vi "בדיקת מתח תפיסה של סליל פיקוד ללא עומס 4.vi"(8 "error":errorcluster, 11 "Path for Log":path) -> (0 "error out":errorcluster, 1 "מצב ממסר פתוח/סגור":bool, 2 "מתח סגירת הממסר":dbl format="%.4f", 3 "מתח מוצא מהספק":dbl format="%.4f", 5 "resultUserPrompt":bool)   [LabVIEW 2015]
uses:
  <vilib>/DAQmx/write.llb/DAQmx Write (Digital Bool 1Line 1Point).vi
  <vilib>/DAQmx/create/channels.llb/DAQmx Create Channel (DO-Digital Output).vi
  <vilib>/DAQmx/miscellaneous.llb/DAQmx Fill In Error Info.vi
panel:
  out "progress":dbl(slide) scale=0.0..36.0
  out "error IO DMM":errorcluster
  in  "Stop Button":bool
  # "Right-Click to\nexplain error"
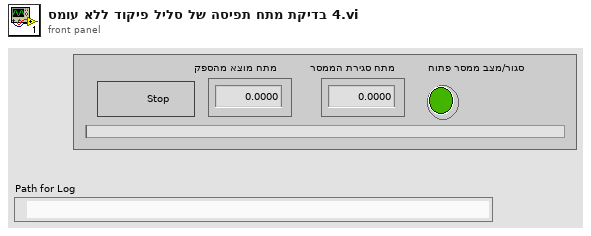
[diagram p1: front panel]
types:
  T1 = enum32{"Invalid", "Standard", "Closed", "Hidden", "Minimized", "Maximized"}
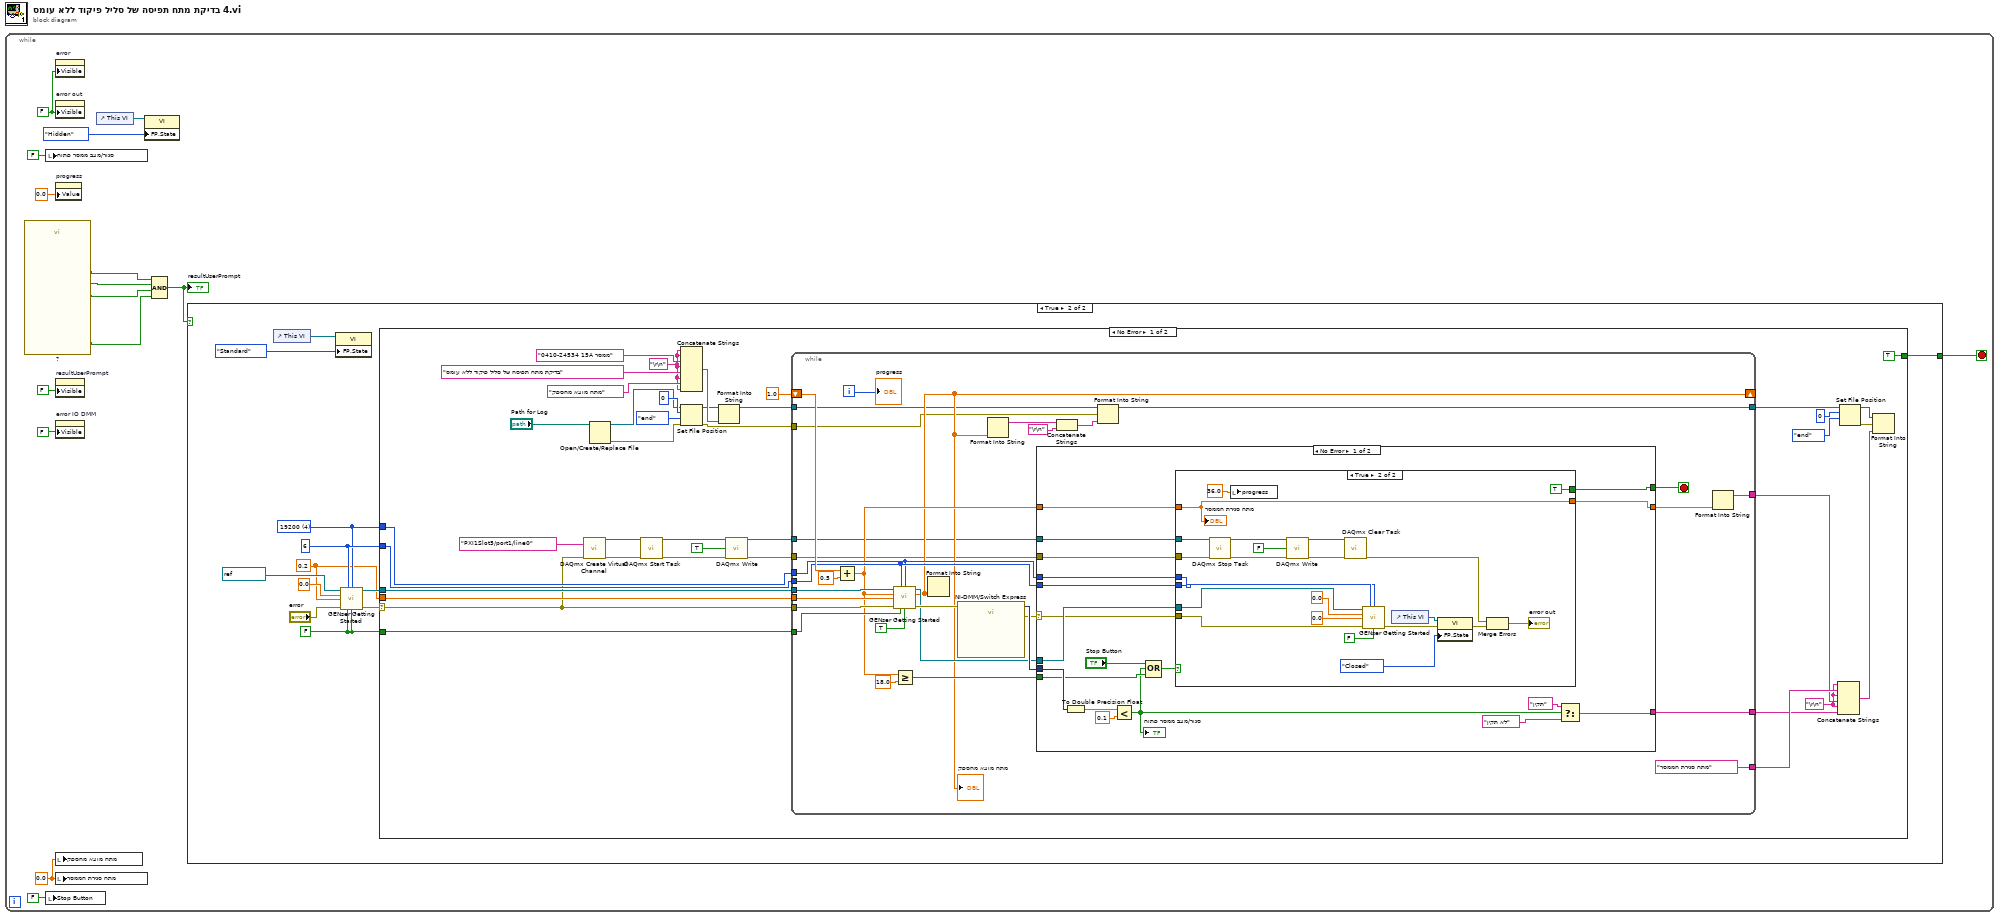
[diagram p0: block diagram]
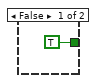
[diagram p2: hidden frame]
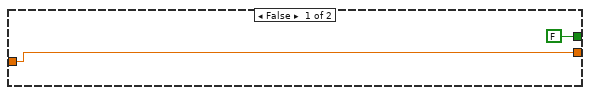
[diagram p3: hidden frame]
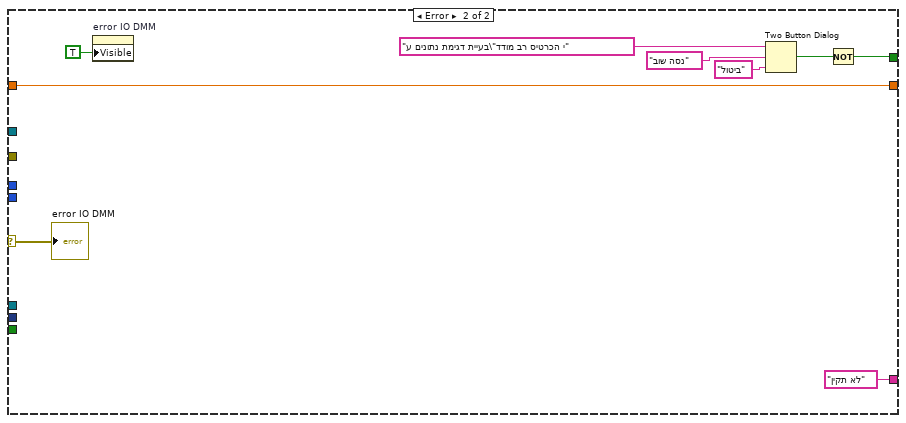
[diagram p4: hidden frame]
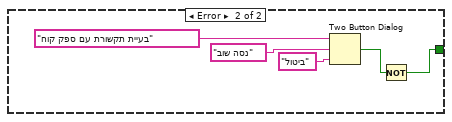
[diagram p5: hidden frame]
diagram:
  n1 = while {
    stop <- w1 stop-if-true
    w7 = FALSE ("Visible")
    w10 = 0.0 ("signals out")
    n2 = call "?"() -> ("הדקי הרב מודד"=w2:bool, "(מגע שלילי (מעטפת"=w3:bool, "A מגע חיובי"=w4:bool, "OK"=w5:bool)  [unwired: 15 in, 1 out]
    n3 = local write "מצב ממסר פתוח/סגור"(FALSE ("מגע סגור")) -> ()
    n4 = local write "Stop Button"(FALSE ("Reset (T)")) -> ()
    n5 = property on="error" class="Clust (strict)"("Visible"=w7) -> ()  [unwired: 2 in, 2 out]
    n6 = property on="error out" class="Clust (strict)"("Visible"=w7) -> ()  [unwired: 2 in, 2 out]
    n7 = property on="progress" class="Slide (strict)"("Value"=0.0 ("progress")) -> ()  [unwired: 2 in, 2 out]
    n8 = property on="resultUserPrompt" class="Bool (strict)"("Visible"=FALSE) -> ()  [unwired: 2 in, 2 out]
    n9 = property on="error IO DMM" class="Clust (strict)"("Visible"=FALSE) -> ()  [unwired: 2 in, 2 out]
    n10 = local write "מתח מוצא מהספק"(w10) -> ()
    n11 = local write "מתח סגירת הממסר"(w10) -> ()
    n12 = control-ref of="This VI"() -> (w9:refnum<vi>)
    n13 = property class="VI"(reference=w9, "FP.State"=T1."Hidden" ("Front Panel Window:State")) -> ()  [unwired: 1 in, 2 out]
    n14 = Compound Arithmetic op=AND(w5, w4, w3, w2) -> (w15:bool)
    "resultUserPrompt" <- w15
    n15 = case shown="True" w15 {
      tunnel: [TRUE ("T button?") w22] -> w1
      frame False {
      }
      frame True {
        w21 = FALSE ("Output On (T)")
        w26 = u16 4 items=["1200", "2400", "4800", "9600", "19200"] ("BAUD")
        w27 = i16 6 ("GEN Addr")
        w23 = 0.2 ("Current Limit")
        n16 = control-ref of="This VI"() -> (w19:refnum<vi>)
        n17 = property class="VI"(reference=w19, "FP.State"=T1."Standard" ("Front Panel Window:State")) -> ()  [unwired: 1 in, 2 out]
        n18 = call "GENser Getting Started.vi"("VISA"=refnum<visa-resource-name> "COM6", "GEN Addr"=w27, "BAUD"=w26, "Voltage Limit"=0.0, "Current Limit"=w23, "error"="error", "Reset (T)"=w21, "Output On (T)"=w21) -> ("VISA out"=w28:refnum<visa-resource-name>, "error out"=w18:errorcluster)  [unwired: 4 in, 2 out]
        n19 = case shown="No Error" w18 {
          selector: w18 -> [w29 _]
          tunnel: w28 -> [w67 _]
          tunnel: w27 -> [w66 _]
          tunnel: w26 -> [w65 _]
          tunnel: w21 -> [w64 _]
          tunnel: w23 -> [w63 _]
          tunnel: [TRUE w152] -> w22
          frame No Error {
            w38 = "\r\n"
            w57 = "\r\n"
            n20 = call-poly <vilib>:"DAQmx Create Virtual Channel.vi"("lines"=tag "PXI1Slot5/port1/line0", "error in"=w29) -> ("task out"=w36:refnum<k21>, "error out"=w37:errorcluster)  [unwired: 12 in]
            n21 = Open/Create/Replace File(file path (use dialog)="Path for Log") -> (refnum out=w48:refnum<file>, error out=w47:errorcluster)  [unwired: 5 in, 1 out]
            n22 = call <vilib>:"DAQmx Start Task.vi"("task/channels in"=w36, "error in"=w37) -> ("task out"=w33:refnum<k21>, "error out"=w32:errorcluster)  [unwired: 12 in]
            n23 = Concatenate Strings(w38, w38, "0410-24534 15A ממסר", w38, "בדיקת מתח תפיסה של סליל פיקוד ללא עומס", w38, "מתח מוצא מהספק", w38) -> (w44:string)
            n24 = Set File Position(offset (in bytes) (0)=i64 0, refnum=w48, from (0:start)=enum16{"start", "end", "current"}."end", error in=w47) -> (refnum out=w40:refnum<file>, error out=w45:errorcluster)
            n25 = Format Into String(initial string=w40, w44) -> (resulting string=w39:refnum<file>)  [unwired: 2 in, 1 out]
            n26 = call-poly <vilib>:"DAQmx Write.vi"("task/channels in"=w33, "data"=TRUE, "error in"=w32) -> ("task out"=w31:refnum<k21>, "error out"=w30:errorcluster)  [unwired: 10 in, 1 out]
            n27 = while {
              tunnel: w67 -> [w87]
              tunnel: w29 -> [w98]
              tunnel: w66 -> [w89]
              tunnel: w65 -> [w88]
              tunnel: w64 -> [w97]
              tunnel: w63 -> [w95]
              shift-right: [w79] -> _
              shift-left: 1.0 ("y") -> [w93]
              tunnel: ["מתח סגירת הממסר"] -> w60
              tunnel: [w77] -> w59
              tunnel: [w76] -> w58
              tunnel: [w73] -> w56
              tunnel: w39 -> [w72]
              tunnel: w45 -> [w71]
              tunnel: w31 -> [w69]
              tunnel: w30 -> [w68]
              i -> [w80]
              stop <- w90 stop-if-true
              n28 = Add(x=w93, y=0.5) -> (x+y=w81:dbl)
              n29 = call "GENser Getting Started.vi"("VISA"=w87, "GEN Addr"=w89, "BAUD"=w88, "Voltage Limit"=w81, "Current Limit"=w95, "error"=w98, "Reset (T)"=w97, "Output On (T)"=TRUE) -> ("VISA out"=w86:refnum<visa-resource-name>, "Output Voltage"=w79:dbl, "error out"=w92:errorcluster)  [unwired: 4 in, 1 out]
              "מתח מוצא מהספק" <- w79
              n30 = Greater Or Equal?(x=w81, y=18.0) -> (x >= y?=w84:bool)
              n31 = Format Into String(w79) -> ()  [unwired: 3 in, 2 out]
              n32 = call "NI-DMM/Switch Express"("error in"=w92) -> ("signals out"=w91:dynamicdata, "error out"=w83:errorcluster)  [unwired: 16 in, 1 out]
              n33 = Format Into String(w79) -> (resulting string=w74:string)  [unwired: 3 in, 1 out]
              n34 = case shown="No Error" w83 {
                selector: w83 -> [w109 w151]
                tunnel: w91 -> [w117 _]
                tunnel: [w106 w143] -> w90
                tunnel: w89 -> [w114 _]
                tunnel: w88 -> [w113 _]
                tunnel: w86 -> [w112 _]
                tunnel: w84 -> [w111 _]
                tunnel: w81 -> [w110 w146]
                tunnel: [w105 w146] -> w82
                tunnel: [w102 "לא תקין"] -> w76
                tunnel: w69 -> [w100 _]
                tunnel: w68 -> [w99 _]
                frame No Error {
                  n35 = To Double Precision Float(number=w117) -> (double precision float=w108:dbl)
                  n36 = Less?(x=w108, y=0.1) -> (x < y?=w101:bool)
                  "מצב ממסר פתוח/סגור" <- w101
                  n37 = Compound Arithmetic op=OR("Stop Button", w101, w111) -> (w116:bool)
                  n38 = case shown="True" w116 {
                    tunnel: [FALSE TRUE] -> w106
                    tunnel: w114 -> [_ w142]
                    tunnel: w113 -> [_ w141]
                    tunnel: w112 -> [_ w140]
                    tunnel: w109 -> [_ w137]
                    tunnel: w110 -> [w118 w132]
                    tunnel: [w118 w132] -> w105
                    tunnel: w100 -> [_ w122]
                    tunnel: w99 -> [_ w121]
                    frame False {
                    }
                    frame True {
                      n39 = call <vilib>:"DAQmx Stop Task.vi"("task/channels in"=w122, "error in"=w121) -> ("task out"=w130:refnum<k21>, "error out"=w128:errorcluster)  [unwired: 12 in]
                      n40 = local write "progress"(36.0 ("progress")) -> ()
                      n41 = call-poly <vilib>:"DAQmx Write.vi"("task/channels in"=w130, "data"=FALSE, "error in"=w128) -> ("task out"=w127:refnum<k21>, "error out"=w126:errorcluster)  [unwired: 10 in, 1 out]
                      n42 = call <vilib>:"DAQmx Clear Task.vi"("task in"=w127, "error in"=w126) -> ("error out"=w123:errorcluster)  [unwired: 13 in]
                      n43 = call "GENser Getting Started.vi"("VISA"=w140, "GEN Addr"=w142, "BAUD"=w141, "Voltage Limit"=0.0, "Current Limit"=0.0, "error"=w137, "Output On (T)"=FALSE) -> ("error out"=w120:errorcluster)  [unwired: 5 in, 3 out]
                      n44 = control-ref of="This VI"() -> (w134:refnum<vi>)
                      n45 = property class="VI"(reference=w134, error in=w120, "FP.State"=T1."Closed" ("Front Panel Window:State")) -> (error out=w124:errorcluster)  [unwired: 1 out]
                      n46 = Merge Errors(w123, w124) -> (→"error out":errorcluster)
                      "מתח סגירת הממסר" <- w132
                    }
                  }
                  n47 = Select(t="תקין", s=w101, f="לא תקין") -> (s? t:f=w102:string)
                }
                frame Error {
                  n48 = property on="error IO DMM" class="Clust (strict)"("Visible"=TRUE) -> ()  [unwired: 2 in, 2 out]
                  n49 = Two Button Dialog(message="בעיית דגימת נתונים ע\"י הכרטיס רב מודד", 1:"ביטול" ("F button name (\"Cancel\")"), 2:"נסה שוב" ("T button name (\"OK\")")) -> (T button?=w144:bool)
                  n50 = Not(x=w144) -> (.not. x?=w143:bool)
                  "error IO DMM" <- w151
                }
              }
              n51 = Concatenate Strings(w74, "\r\n") -> (w70:string)
              n52 = Format Into String(initial string=w72, error in=w71, w70) -> (resulting string=w73:refnum<file>)  [unwired: 1 in, 1 out]
              n53 = Format Into String(w82) -> (resulting string=w77:string)  [unwired: 3 in, 1 out]
              "progress" <- w80
            }
            n54 = Concatenate Strings(w57, w60, w57, w59, w57, w58) -> (w51:string)
            n55 = Set File Position(offset (in bytes) (0)=i64 0, refnum=w56, from (0:start)=enum16{"start", "end", "current"}."end") -> (refnum out=w53:refnum<file>, error out=w52:errorcluster)  [unwired: 1 in]
            n56 = Format Into String(initial string=w53, error in=w52, w51) -> ()  [unwired: 1 in, 2 out]
          }
          frame Error {
            n57 = Two Button Dialog(message="בעיית תקשורת עם ספק קוח", 1:"ביטול" ("F button name (\"Cancel\")"), 2:"נסה שוב" ("T button name (\"OK\")")) -> (T button?=w153:bool)
            n58 = Not(x=w153) -> (.not. x?=w152:bool)
          }
        }
      }
    }
  }
